vi "XControl with User Events Uninit.vi"(2 "Container State":T1, 3 "Display State":T2) -> ()   [LabVIEW 2009, in "XControlUserEvents.xctl"]
doc: "Demonstration of an XControl.\n\nAAL 9/09"
uses:
  XControlUserEvents.xctl
  XControl with User Events State.ctl
  <vilib>/_xctls/Container State.ctl
  <vilib>/_xctls/XControlSupport.lvlib
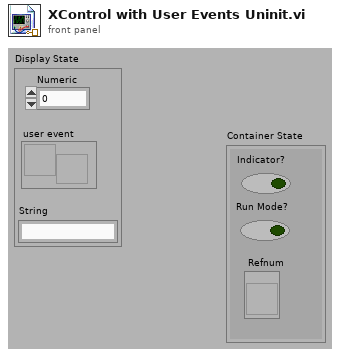
[diagram p1: front panel]
types:
  T1 = typedef "XControlSupport.lvlib/Container State.ctl" = cluster{"Indicator?":bool, "Run Mode?":bool, " Refnum":refnum<vi>}
  T2 = typedef "XControlUserEvents.xctl/XControl with User Events State.ctl" = cluster{"Numeric":dbl, "user event":refnum<user-event>, "String":string}
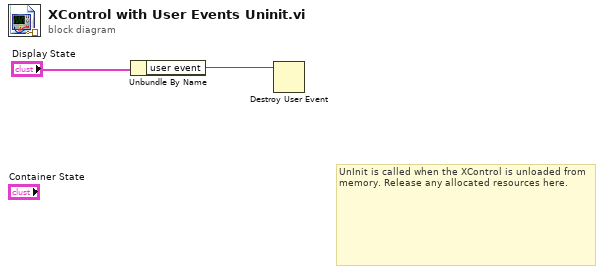
[diagram p0: block diagram]
diagram:
  # "UnInit is called when the XControl is unloaded from memory. Release any allocated resources here."
  n1 = Unbundle By Name("Display State") -> ("user event"=w1:refnum<user-event>)
  n2 = Destroy User Event(user event=w1) -> ()  [unwired: 1 in, 1 out]
